vi "Build Display Selections.vi"(6 "Write":bool=TRUE, 7 "ID Prefix":string, 8 "Owner":i32, 9 "Sub Items":T2[](array[typedef]), 10 "Item Name":string, 11 "Type":variant) -> (3 "Array":T1[](array[typedef]))   [LabVIEW 2015, in "Read-Write-Signals.xnode"]
uses:
  Read-Write-Signals.xnode
  Read-Write-Signals Sub Item.ctl
  Read-Write-Signals Sub Item Type.ctl
  Read-Write-Signals Display Selection.ctl
  <vilib>/Utility/Data Type/NI_Data Type.lvlib
  <vilib>/Erdos Miller/LV-Scripting/LV-Scripting.lvlib
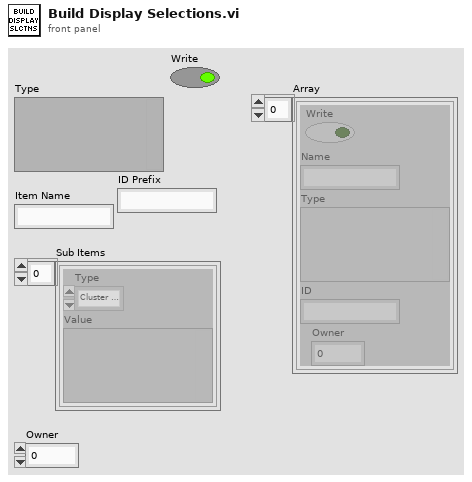
[diagram p1: front panel]
types:
  T1 = typedef "Read-Write-Signals Display Selection.ctl" = cluster{"Write":bool, "Name":string, "Type":variant, "ID":string, "Owner":i32}
  T2 = typedef "Read-Write-Signals Sub Item.ctl" = cluster{"Type":T3, "Value":variant}
  T3 = typedef "Read-Write-Signals Sub Item Type.ctl" = enum8{"Cluster Element", "Array Element", "Subarray"}
  T4 = typedef "NI_Data Type.lvlib/Memory Info.ctl" = cluster{"Type":T5, "Size":u32}
  T5 = typedef "NI_Data Type.lvlib/Memory Type.ctl" = enum16{"Variable", "Fixed", "Bounded"}
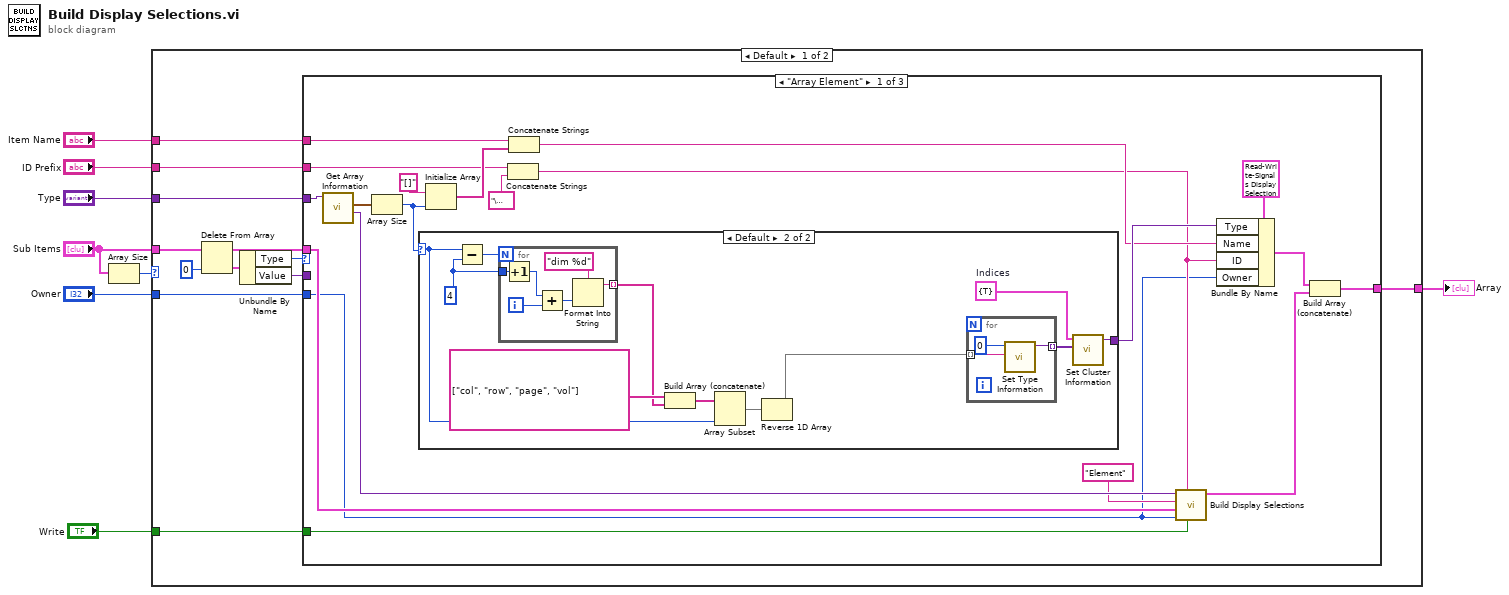
[diagram p0: block diagram]
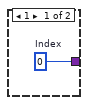
[diagram p2: hidden frame]
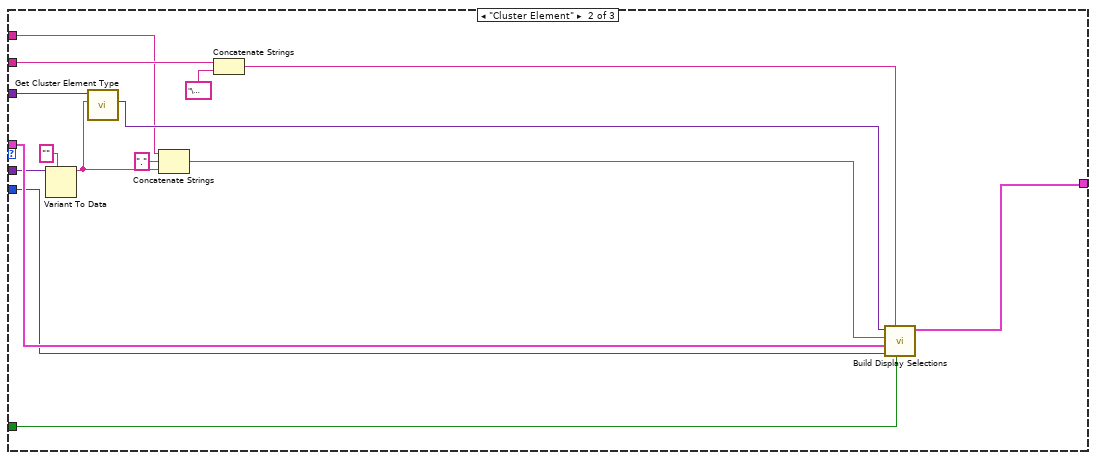
[diagram p3: hidden frame]
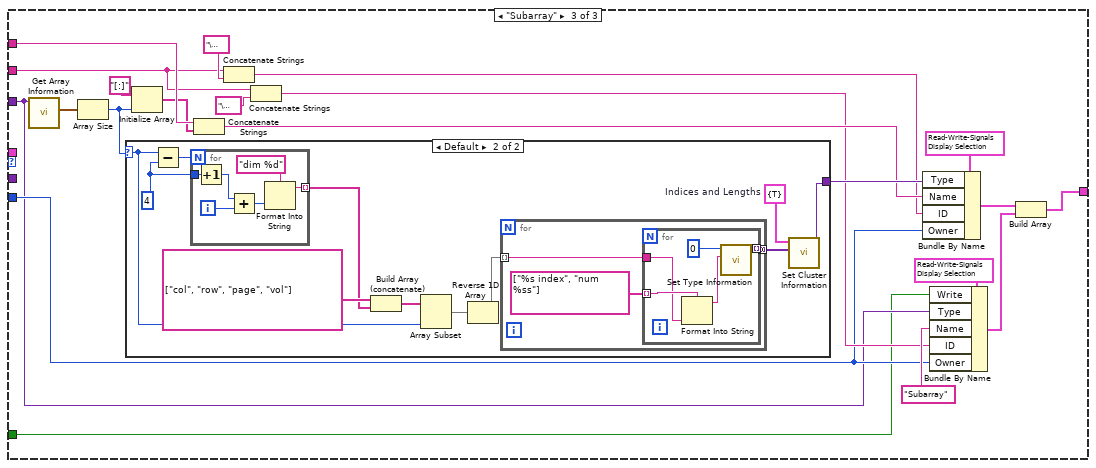
[diagram p4: hidden frame]
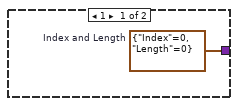
[diagram p5: hidden frame]
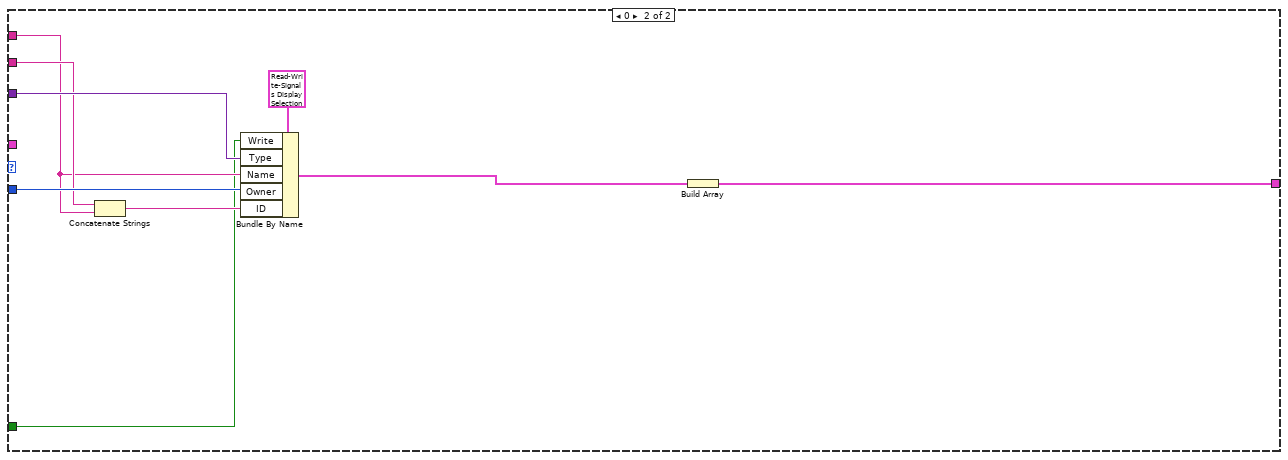
[diagram p6: hidden frame]
diagram:
  n1 = Array Size(array="Sub Items") -> (size(s)=w8:i32)
  n2 = case shown="Default" w8 {
    tunnel: "Item Name" -> [w14 w125]
    tunnel: "Type" -> [w15 w131]
    tunnel: "Owner" -> [w12 w127]
    tunnel: [w10 w129] -> w4
    tunnel: "Sub Items" -> [w20 _]
    tunnel: "ID Prefix" -> [w13 w126]
    tunnel: "Write" -> [w9 w124]
    frame Default {
      n3 = Delete From Array(array=w20, index=0) -> (deleted portion=w18:T2, array with subset deleted=w11:T2[])  [unwired: 1 in]
      n4 = Unbundle By Name(w18) -> ("Type"=w17:T3, "Value"=w16:variant)
      n5 = case shown="\"Array Element\"" w17 {
        tunnel: w16 -> [_ w70 _]
        tunnel: w15 -> [w40 w71 w78]
        tunnel: w14 -> [w37 w67 w95]
        tunnel: w13 -> [w31 w76 w83]
        tunnel: w12 -> [w25 w73 w81]
        tunnel: w11 -> [w26 w74 _]
        tunnel: [w22 w63 w87] -> w10
        tunnel: w9 -> [w21 w62 w77]
        frame "Array Element" {
          n6 = call <vilib>:"Get Array Information.vi"("Variant"=w40) -> ("Array Element Data Type"=w29:variant, "Array Lengths"=w39:T4[])  [unwired: 7 in, 2 out]
          n7 = Array Size(array=w39) -> (size(s)=w35:i32)
          n8 = case shown="Default" w35 {
            selector: w35 -> [_ w42]
            tunnel: [w41 w46] -> w33
            frame 1 {
              w41 = 0  # Index
            }
            frame Default {
              w43 = cluster{bool} {TRUE}  # Indices
              w51 = 4 ("y")
              n9 = Subtract(x=w42, y=w51) -> (x-y=w52:i32)
              n10 = for {
                N: w52 -> [_]
                tunnel: w51 -> [w60]
                tunnel: [w57] -> w49 mode=indexing
                i -> [w61]
                n11 = Increment(x=w60) -> (x+1=w56:i32)
                n12 = Add(x=w56, y=w61) -> (x+y=w59:i32)
                n13 = Format Into String(format string="dim %d", w59) -> (resulting string=w57:string)  [unwired: 2 in, 1 out]
              }
              n14 = Build Array (concatenate)(string[] ["col", "row", "page", "vol"] ("Names"), w49) -> (w48:string[])
              n15 = Array Subset(array=w48, length=w42) -> (w47:string[])  [unwired: 1 in]
              n16 = Reverse 1D Array(array=w47) -> (reversed array=w45:string[])
              n17 = for {
                tunnel: w45 -> [w54] mode=indexing
                tunnel: [w53] -> w44 mode=indexing
                n18 = call <vilib>:"Set Type Information.vi"("Name"=w54, "Variant in"=0) -> ("Variant out"=w53:variant)  [unwired: 8 in, 1 out]
              }
              n19 = call <vilib>:"Set Cluster Information.vi"("Cluster Elements"=w44, "Variant in"=w43) -> ("Variant out"=w46:variant)  [unwired: 8 in, 1 out]
            }
          }
          n20 = Initialize Array("[]", w35) -> (w36:string[])
          n21 = Concatenate Strings(w31, "\u0001" ("string")) -> (w28:string)
          n22 = Concatenate Strings(w37, w36) -> (w32:string)
          n23 = call "Build Display Selections.vi"("Write"=w21, "ID Prefix"=w28, "Owner"=w25, "Sub Items"=w26, "Item Name"="Element", "Type"=w29) -> ("Array"=w24:T1[])  [unwired: 5 in]
          n24 = Bundle By Name(cluster=T1 {"Write"=TRUE, "Name"="", "Type"=variant, "ID"="", "Owner"=0} ("Selection"), "Type"=w33, "Name"=w32, "ID"=w28, "Owner"=w25) -> (w23:T1)
          n25 = Build Array (concatenate)(w23, w24) -> (w22:T1[])
        }
        frame "Cluster Element" {
          n26 = Variant To Data(type="", Variant=w70) -> (data=w65:string)  [unwired: 1 in, 1 out]
          n27 = call <vilib>:"Get Cluster Element Type.vi"("Element Name"=w65, "Cluster in"=w71) -> ("Type"=w68:variant)  [unwired: 7 in, 2 out]
          n28 = Concatenate Strings(w67, "." ("string"), w65) -> (w64:string)
          n29 = Concatenate Strings(w76, "\u0000" ("string")) -> (w72:string)
          n30 = call "Build Display Selections.vi"("Write"=w62, "ID Prefix"=w72, "Owner"=w73, "Sub Items"=w74, "Item Name"=w64, "Type"=w68) -> ("Array"=w63:T1[])  [unwired: 5 in]
        }
        frame "Subarray" {
          n31 = call <vilib>:"Get Array Information.vi"("Variant"=w78) -> ("Array Lengths"=w97:T4[])  [unwired: 7 in, 3 out]
          n32 = Array Size(array=w97) -> (size(s)=w93:i32)
          n33 = case shown="Default" w93 {
            selector: w93 -> [_ w99]
            tunnel: [w98 w100] -> w91
            frame 1 {
              w98 = cluster{"Index":i32, "Length":i32} {"Index"=0, "Length"=0}  # Index and Length
            }
            frame Default {
              w101 = cluster{bool} {TRUE}  # Indices and Lengths
              w108 = 4 ("y")
              n34 = Subtract(x=w99, y=w108) -> (x-y=w109:i32)
              n35 = for {
                N: w109 -> [_]
                tunnel: w108 -> [w122]
                tunnel: [w119] -> w106 mode=indexing
                i -> [w123]
                n36 = Increment(x=w122) -> (x+1=w118:i32)
                n37 = Add(x=w118, y=w123) -> (x+y=w121:i32)
                n38 = Format Into String(format string="dim %d", w121) -> (resulting string=w119:string)  [unwired: 2 in, 1 out]
              }
              n39 = Build Array (concatenate)(string[] ["col", "row", "page", "vol"] ("Names"), w106) -> (w105:string[])
              n40 = Array Subset(array=w105, length=w99) -> (w104:string[])  [unwired: 1 in]
              n41 = Reverse 1D Array(array=w104) -> (reversed array=w103:string[])
              n42 = for {
                tunnel: w103 -> [w111] mode=indexing
                tunnel: [w112] -> w102 mode=concatenating
                n43 = for {
                  tunnel: [w116] -> w112 mode=indexing
                  tunnel: w111 -> [w114]
                  tunnel: string[] ["%s index", "num %ss"] ("Names") -> [w115] mode=indexing
                  n44 = Format Into String(format string=w115, w114) -> (resulting string=w113:string)  [unwired: 2 in, 1 out]
                  n45 = call <vilib>:"Set Type Information.vi"("Name"=w113, "Variant in"=0) -> ("Variant out"=w116:variant)  [unwired: 8 in, 1 out]
                }
              }
              n46 = call <vilib>:"Set Cluster Information.vi"("Cluster Elements"=w102, "Variant in"=w101) -> ("Variant out"=w100:variant)  [unwired: 8 in, 1 out]
            }
          }
          n47 = Initialize Array("[:]", w93) -> (w94:string[])
          n48 = Concatenate Strings(w95, w94) -> (w90:string)
          n49 = Concatenate Strings(w83, "\u0002" ("string")) -> (w84:string)
          n50 = Concatenate Strings(w83, "\u0003" ("string")) -> (w82:string)
          n51 = Bundle By Name(cluster=T1 {"Write"=TRUE, "Name"="", "Type"=variant, "ID"="", "Owner"=0} ("Selection"), "Type"=w91, "Name"=w90, "ID"=w84, "Owner"=w81) -> (w88:T1)
          n52 = Bundle By Name(cluster=T1 {"Write"=FALSE, "Name"="", "Type"=variant, "ID"="", "Owner"=0} ("Selection"), "Write"=w77, "Type"=w78, "Name"="Subarray", "ID"=w82, "Owner"=w81) -> (w79:T1)
          n53 = Build Array(w88, w79) -> (w87:T1[])
        }
      }
    }
    frame 0 {
      n54 = Concatenate Strings(w126, w125) -> (w128:string)
      n55 = Bundle By Name(cluster=T1 {"Write"=FALSE, "Name"="", "Type"=variant, "ID"="", "Owner"=0} ("Selection"), "Write"=w124, "Type"=w131, "Name"=w125, "Owner"=w127, "ID"=w128) -> (w130:T1)
      n56 = Build Array(w130) -> (w129:T1[])
    }
  }
  "Array" <- w4
